vi "MakeTable.vi"(8 "PlotCounty":string, 11 "TableData":T2(array[cluster])) -> (2 "Strings":T1, 3 "TableOut":string[][](table))   [LabVIEW 2017]
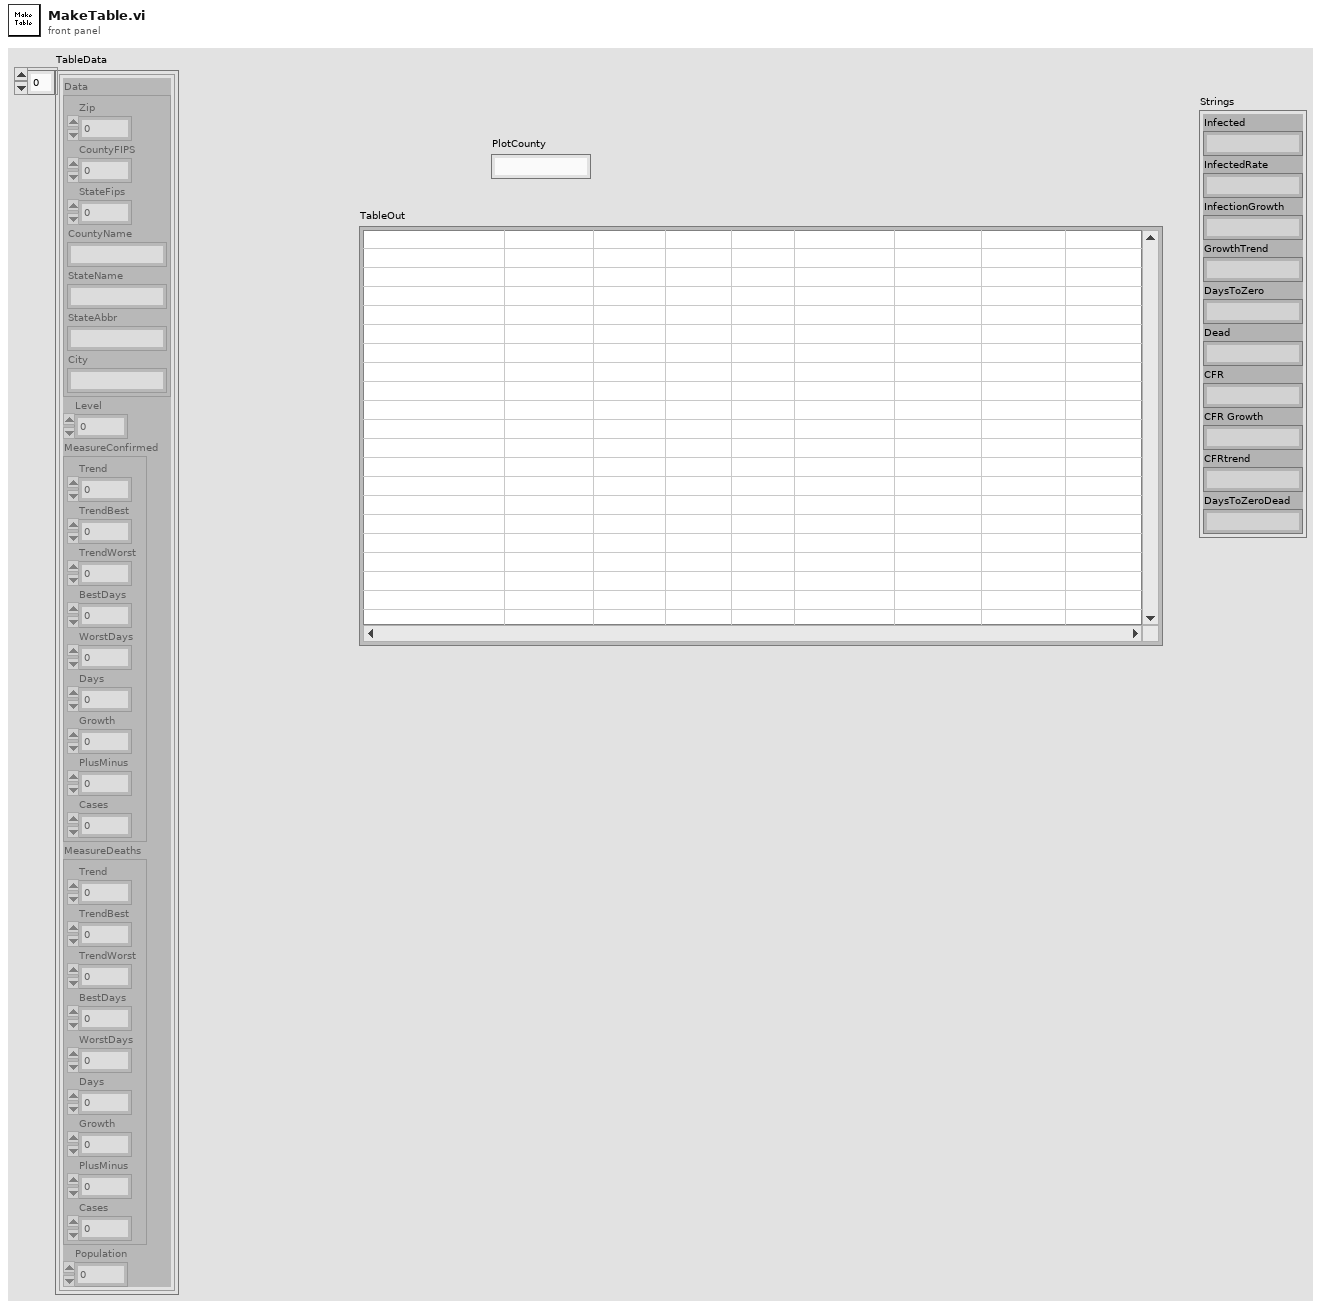
[diagram p1: front panel]
types:
  T1 = cluster{"Infected":string, "InfectedRate":string, "InfectionGrowth":string, "GrowthTrend":string, "DaysToZero":string, "Dead":string, "CFR":string, "CFR Growth":string, "CFRtrend":string, "DaysToZeroDead":string}
  T2 = cluster{"Data":cluster{"Zip":i32, "CountyFIPS":i32, "StateFips":i32, "CountyName":string, "StateName":string, "StateAbbr":string, "City":string}, "Level":u16, "MeasureConfirmed":cluster{"Trend":dbl, "TrendBest":dbl, "TrendWorst":dbl, "BestDays":dbl, "WorstDays":dbl, "Days":dbl, "Growth":dbl, "PlusMinus":dbl, "Cases":i32}, "MeasureDeaths":cluster{"Trend":dbl, "TrendBest":dbl, "TrendWorst":dbl, "BestDays":dbl, "WorstDays":dbl, "Days":dbl, "Growth":dbl, "PlusMinus":dbl, "Cases":i32}, "Population":i32}[]
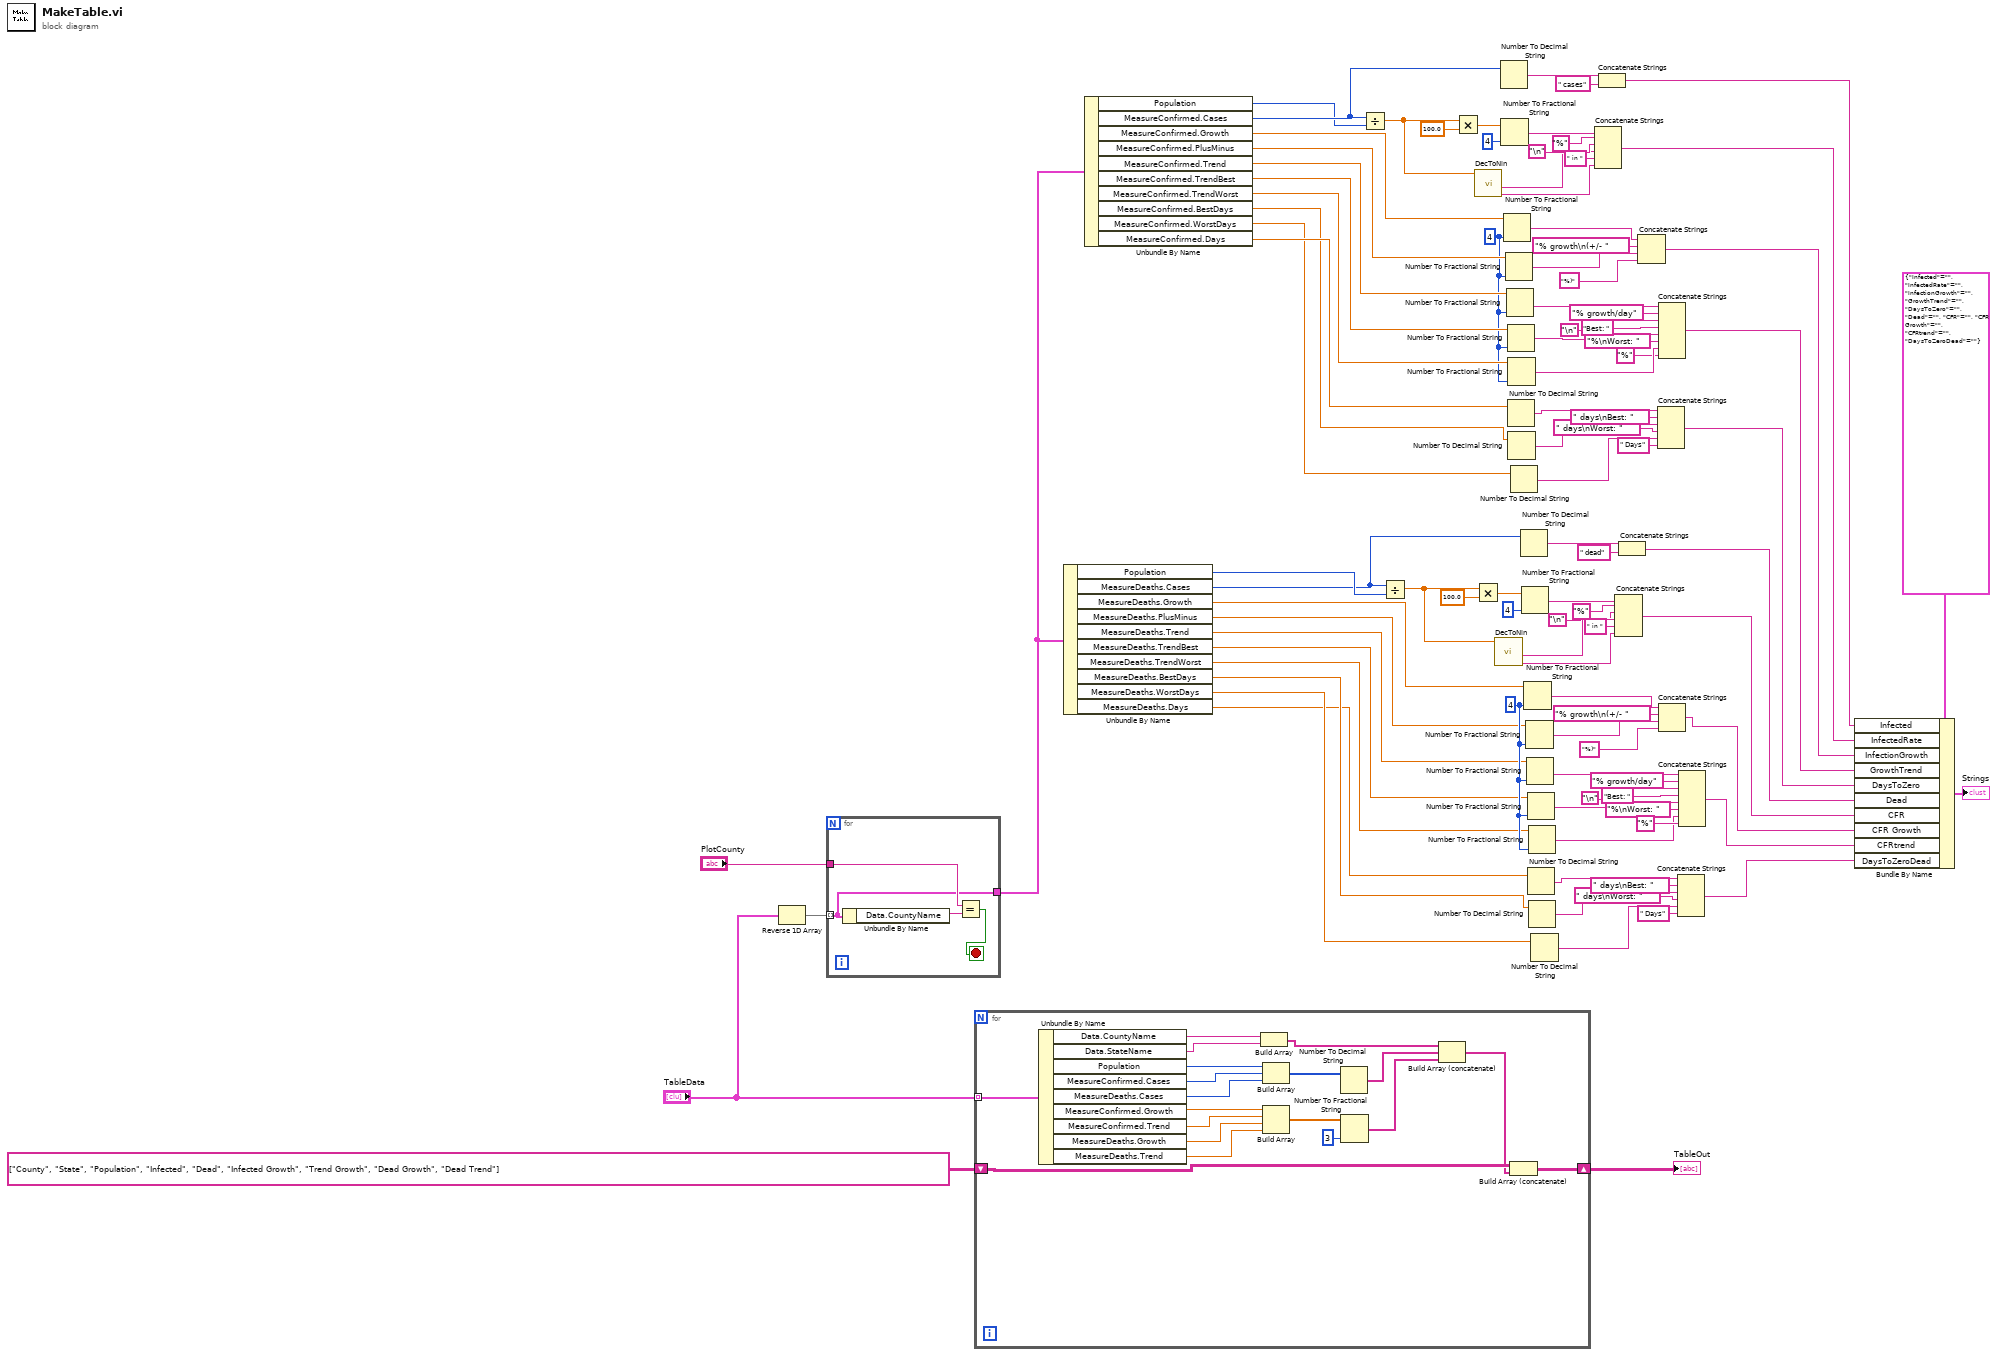
[diagram p0: block diagram]
diagram:
  w43 = i16 4 ("precision (6)")
  w65 = i16 4 ("precision (6)")
  n1 = Reverse 1D Array(array="TableData") -> (reversed array=w1:T2)
  n2 = for {
    tunnel: "PlotCounty" -> [w103]
    tunnel: w1 -> [w101] mode=indexing
    tunnel: [w101] -> w3
    stop <- w102 stop-if-true
    n3 = Unbundle By Name(w101) -> ("Data.CountyName"=w104:string)
    n4 = Equal?(x=w103, y=w104) -> (x = y?=w102:bool)
  }
  n5 = for {
    tunnel: "TableData" -> [w123] mode=indexing
    shift-right: [w106] -> w99
    shift-left: string[][] [["County", "State", "Population", "Infected", "Dead", "Infected Growth", "Trend Growth", "Dead Growth", "Dead Trend"]] ("TableOut") -> [w107]
    n6 = Unbundle By Name(w123) -> ("Data.CountyName"=w122:string, "Data.StateName"=w121:string, "Population"=w120:i32, "MeasureConfirmed.Cases"=w119:i32, "MeasureDeaths.Cases"=w118:i32, "MeasureConfirmed.Growth"=w116:dbl, "MeasureConfirmed.Trend"=w115:dbl, "MeasureDeaths.Growth"=w114:dbl, "MeasureDeaths.Trend"=w113:dbl)
    n7 = Build Array(w122, w121) -> (w110:string[])
    n8 = Build Array(w120, w119, w118) -> (w117:i32[])
    n9 = Build Array(w116, w115, w114, w113) -> (w112:dbl[])
    n10 = Number To Decimal String(number=w117) -> (decimal integer string=w109:string[])  [unwired: 1 in]
    n11 = Number To Fractional String(number=w112, precision (6)=i16 3) -> (F-format string=w108:string[])  [unwired: 2 in]
    n12 = Build Array (concatenate)(w110, w109, w108) -> (w105:string[])
    n13 = Build Array (concatenate)(w107, w105) -> (w106:string[][])
  }
  "TableOut" <- w99
  n14 = Unbundle By Name(w3) -> ("Population"=w20:i32, "MeasureDeaths.Cases"=w19:i32, "MeasureDeaths.Growth"=w18:dbl, "MeasureDeaths.PlusMinus"=w17:dbl, "MeasureDeaths.Trend"=w16:dbl, "MeasureDeaths.TrendBest"=w15:dbl, "MeasureDeaths.TrendWorst"=w14:dbl, "MeasureDeaths.BestDays"=w13:dbl, "MeasureDeaths.WorstDays"=w12:dbl, "MeasureDeaths.Days"=w11:dbl)
  n15 = Unbundle By Name(w3) -> ("Population"=w93:i32, "MeasureConfirmed.Cases"=w94:i32, "MeasureConfirmed.Growth"=w81:dbl, "MeasureConfirmed.PlusMinus"=w78:dbl, "MeasureConfirmed.Trend"=w74:dbl, "MeasureConfirmed.TrendBest"=w70:dbl, "MeasureConfirmed.TrendWorst"=w66:dbl, "MeasureConfirmed.BestDays"=w58:dbl, "MeasureConfirmed.WorstDays"=w55:dbl, "MeasureConfirmed.Days"=w61:dbl)
  n16 = Divide(x=w94, y=w93) -> (x/y=w87:dbl)
  n17 = Divide(x=w19, y=w20) -> (x/y=w28:dbl)
  n18 = Multiply(x=w87, y=100.0) -> (x*y=w89:dbl)
  n19 = call "DecToNin.vi"("Decimal"=w87) -> ("10^x"=w83:string, "Nin"=w85:string)  [unwired: 7 in, 2 out]
  n20 = Multiply(x=w28, y=100.0) -> (x*y=w26:dbl)
  n21 = call "DecToNin.vi"("Decimal"=w28) -> ("10^x"=w32:string, "Nin"=w30:string)  [unwired: 7 in, 2 out]
  n22 = Number To Decimal String(number=w94) -> (decimal integer string=w97:string)  [unwired: 1 in]
  n23 = Number To Fractional String(number=w89, precision (6)=i16 4) -> (F-format string=w92:string)  [unwired: 2 in]
  n24 = Number To Fractional String(number=w81, precision (6)=w65) -> (F-format string=w80:string)  [unwired: 2 in]
  n25 = Number To Fractional String(number=w78, precision (6)=w65) -> (F-format string=w77:string)  [unwired: 2 in]
  n26 = Number To Fractional String(number=w74, precision (6)=w65) -> (F-format string=w73:string)  [unwired: 2 in]
  n27 = Number To Fractional String(number=w70, precision (6)=w65) -> (F-format string=w68:string)  [unwired: 2 in]
  n28 = Number To Decimal String(number=w61) -> (decimal integer string=w60:string)  [unwired: 1 in]
  n29 = Number To Fractional String(number=w66, precision (6)=w65) -> (F-format string=w64:string)  [unwired: 2 in]
  n30 = Number To Decimal String(number=w58) -> (decimal integer string=w57:string)  [unwired: 1 in]
  n31 = Number To Decimal String(number=w55) -> (decimal integer string=w54:string)  [unwired: 1 in]
  n32 = Number To Decimal String(number=w19) -> (decimal integer string=w21:string)  [unwired: 1 in]
  n33 = Number To Fractional String(number=w26, precision (6)=i16 4) -> (F-format string=w23:string)  [unwired: 2 in]
  n34 = Number To Fractional String(number=w18, precision (6)=w43) -> (F-format string=w33:string)  [unwired: 2 in]
  n35 = Number To Fractional String(number=w17, precision (6)=w43) -> (F-format string=w35:string)  [unwired: 2 in]
  n36 = Number To Fractional String(number=w16, precision (6)=w43) -> (F-format string=w37:string)  [unwired: 2 in]
  n37 = Number To Fractional String(number=w15, precision (6)=w43) -> (F-format string=w41:string)  [unwired: 2 in]
  n38 = Number To Decimal String(number=w11) -> (decimal integer string=w46:string)  [unwired: 1 in]
  n39 = Number To Fractional String(number=w14, precision (6)=w43) -> (F-format string=w44:string)  [unwired: 2 in]
  n40 = Number To Decimal String(number=w13) -> (decimal integer string=w48:string)  [unwired: 1 in]
  n41 = Number To Decimal String(number=w12) -> (decimal integer string=w50:string)  [unwired: 1 in]
  n42 = Concatenate Strings(w92, "%" ("string"), "\n", w85, " in " ("string"), w83) -> (w82:string)
  n43 = Concatenate Strings(w97, " cases" ("string")) -> (w95:string)
  n44 = Concatenate Strings(w23, "%" ("string"), "\n", w30, " in " ("string"), w32) -> (w9:string)
  n45 = Concatenate Strings(w21, " dead" ("string")) -> (w10:string)
  n46 = Concatenate Strings(w80, "% growth\n(+/- " ("string"), w77, "%)" ("string")) -> (w75:string)
  n47 = Concatenate Strings(w60, " days\nBest: " ("string"), w57, " days\nWorst: " ("string"), w54, " Days" ("string")) -> (w52:string)
  n48 = Concatenate Strings(w73, "% growth/day" ("string"), "\n", "Best: " ("string"), w68, "%\nWorst: " ("string"), w64, "%" ("string")) -> (w62:string)
  n49 = Concatenate Strings(w33, "% growth\n(+/- " ("string"), w35, "%)" ("string")) -> (w8:string)
  n50 = Concatenate Strings(w46, " days\nBest: " ("string"), w48, " days\nWorst: " ("string"), w50, " Days" ("string")) -> (w6:string)
  n51 = Concatenate Strings(w37, "% growth/day" ("string"), "\n", "Best: " ("string"), w41, "%\nWorst: " ("string"), w44, "%" ("string")) -> (w7:string)
  n52 = Bundle By Name(cluster=T1 {"Infected"="", "InfectedRate"="", "InfectionGrowth"="", "GrowthTrend"="", "DaysToZero"="", "Dead"="", "CFR"="", "CFR Growth"="", "CFRtrend"="", "DaysToZeroDead"=""}, "Infected"=w95, "InfectedRate"=w82, "InfectionGrowth"=w75, "GrowthTrend"=w62, "DaysToZero"=w52, "Dead"=w10, "CFR"=w9, "CFR Growth"=w8, "CFRtrend"=w7, "DaysToZeroDead"=w6) -> (→"Strings":T1)
